vi "JsonToAttrMap.vi"(6 "lower case Key?(F)":bool, 7 "Type and Defaults":variant, 8 "error in (no error)":errorcluster, 11 "Json":string) -> (0 "error out":errorcluster, 3 "AttrMap":variant)   [LabVIEW 2019, in "lv-apt-json-file.lvlib"]
uses:
  lv-apt-json-file.lvlib
  <vilib>/Utility/error.llb/Clear Errors.vi
  Remove Comments.vi
  <userlib>/NEVSTOP-Programming-Palette/Configuration/Ini/TextToLines.vi
  <userlib>/NEVSTOP-Programming-Palette/Configuration/Ini/Lines Filter-Annotation.vi
  <userlib>/NEVSTOP-Programming-Palette/Configuration/Ini/LinesToText.vi
  <vilib>/Utility/error.llb/Error Cluster From Error Code.vi
  <vilib>/addons/_JKI.lib/Serialization/JSON/JKI JSON Serialization.lvlib
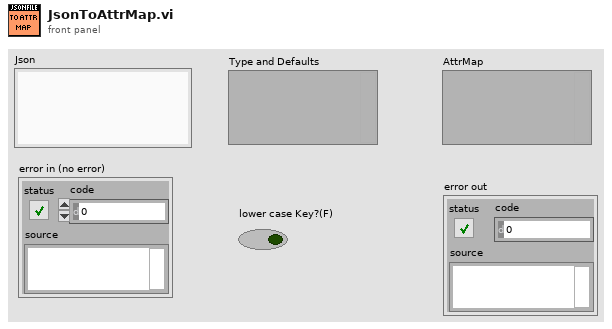
[diagram p1: front panel]
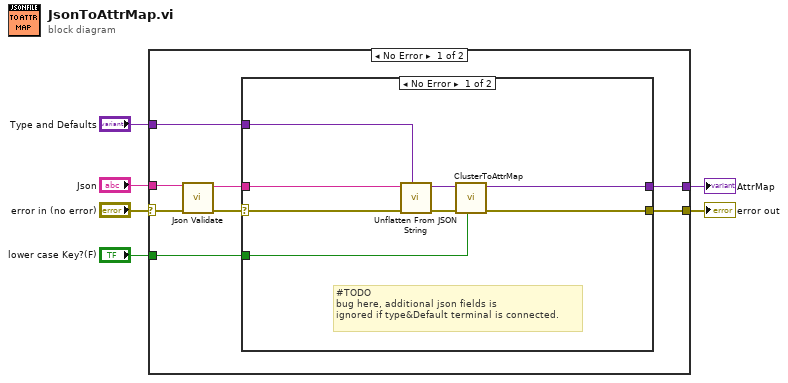
[diagram p0: block diagram]
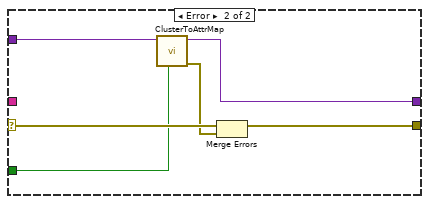
[diagram p2: hidden frame]
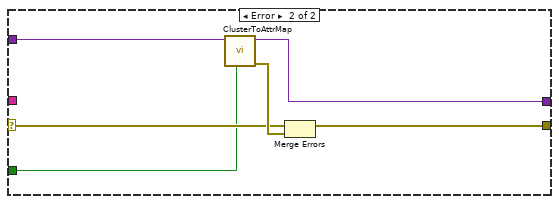
[diagram p3: hidden frame]
diagram:
  n1 = case shown="No Error" "error in (no error)" {
    selector: "error in (no error)" -> [w13 w31]
    tunnel: "Json" -> [w14 _]
    tunnel: "Type and Defaults" -> [w11 w33]
    tunnel: "lower case Key?(F)" -> [w10 w30]
    tunnel: [w9 w29] -> w2
    tunnel: [w8 w32] -> w1
    frame No Error {
      n2 = call "Json Validate.vi"("error in (no error)"=w13, "String"=w14) -> ("error out"=w12:errorcluster, "Json without comments"=w7:string)  [unwired: 6 in, 2 out]
      n3 = case shown="No Error" w12 {
        selector: w12 -> [w16 w28]
        tunnel: w7 -> [w22 _]
        tunnel: w11 -> [w15 w27]
        tunnel: w10 -> [w19 w26]
        tunnel: [w18 w25] -> w9
        tunnel: [w17 w24] -> w8
        frame No Error {
          # "#TODO\nbug here, additional json fields is\nignored if type&Default terminal is connected."
          n4 = call <vilib>:"Unflatten From JSON String.vi"("Type and Defaults"=w15, "error in (no error)"=w16, "JSON String"=w22) -> ("error out"=w20:errorcluster, "Variant"=w21:variant)  [unwired: 7 in]
          n5 = call "ClusterToAttrMap.vi"("lower case Key?(F)"=w19, "error in (no error)"=w20, "data"=w21) -> ("error out"=w18:errorcluster, "AttrMap"=w17:variant)  [unwired: 7 in]
        }
        frame Error {
          n6 = call "ClusterToAttrMap.vi"("lower case Key?(F)"=w26, "data"=w27) -> ("error out"=w23:errorcluster, "AttrMap"=w24:variant)  [unwired: 8 in]
          n7 = Merge Errors(w28, w23) -> (w25:errorcluster)
        }
      }
    }
    frame Error {
      n8 = call "ClusterToAttrMap.vi"("lower case Key?(F)"=w30, "data"=w33) -> ("error out"=w34:errorcluster, "AttrMap"=w32:variant)  [unwired: 8 in]
      n9 = Merge Errors(w31, w34) -> (w29:errorcluster)
    }
  }
  "error out" <- w2
  "AttrMap" <- w1
